vi "Auto_Routine_StraightTwoPieceTRAJ.vi"(8 "error in (no error)":errorcluster) -> (0 "error out":errorcluster)   [LabVIEW 2023]
doc: "Moves from middle of the speaker to the middle note on robot starting line and back \n*****DOES NOT HAVE WAIT AFTER COMPLETE*****\n-Sets arm to speaker Pose\n-Pre rev\n-Waits for arm (to get to speaker shooot pose)\n-Shoots note\n-Waits for box to shoot note\n-Sets arm to floor\n-Runs intake\n-Moves to note\n-Sets arm to speaker pose\n-20 ms wait\n-Goes back to speaker (while waiting for note to intake and pre rev-ing)\n-Waits for arm (to be at speaker shoot pose)\n-Shoots note\n-Waits for shoot to be done \n-Sets arm to floor"
uses:
  Shoulder/ShoulderGetSetpointEnum.ctl
  Trajectory/TrajectoryGlobals.vi
  <vilib>/Rock Robotics/WPI/ThirdParty/JAS_Junk/TrajLib/Trajectory_Library.lvlib
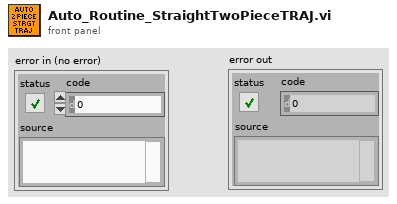
[diagram p1: front panel]
types:
  T1 = typedef "ShoulderGetSetpointEnum.ctl" = enum16{"ShoulderRest", "ShoulderSpeaker", "ShoulderAmp"}
  T2 = typedef "Trajectory_Library.lvlib/TRAJECTORY.ctl" = cluster{"TotalTImeSecs":dbl, "States":T3[]}
  T3 = typedef "Trajectory_Library.lvlib/TRAJ_STATE.ctl" = cluster{"TimeSeconds":dbl, "Velocity":dbl, "Acceleration":dbl, "POSE":T4, "Curvature":dbl}
  T4 = typedef "Trajectory_Library.lvlib/POSE2D.ctl" = cluster{"TRANSLATION":T5, "ROTATION":T6}
  T5 = typedef "Trajectory_Library.lvlib/TRANSLATION2D.ctl" = cluster{"X":dbl, "Y":dbl}
  T6 = typedef "Trajectory_Library.lvlib/ROTATION2D.ctl" = cluster{"VALUE":dbl, "COS":dbl, "SIN":dbl}
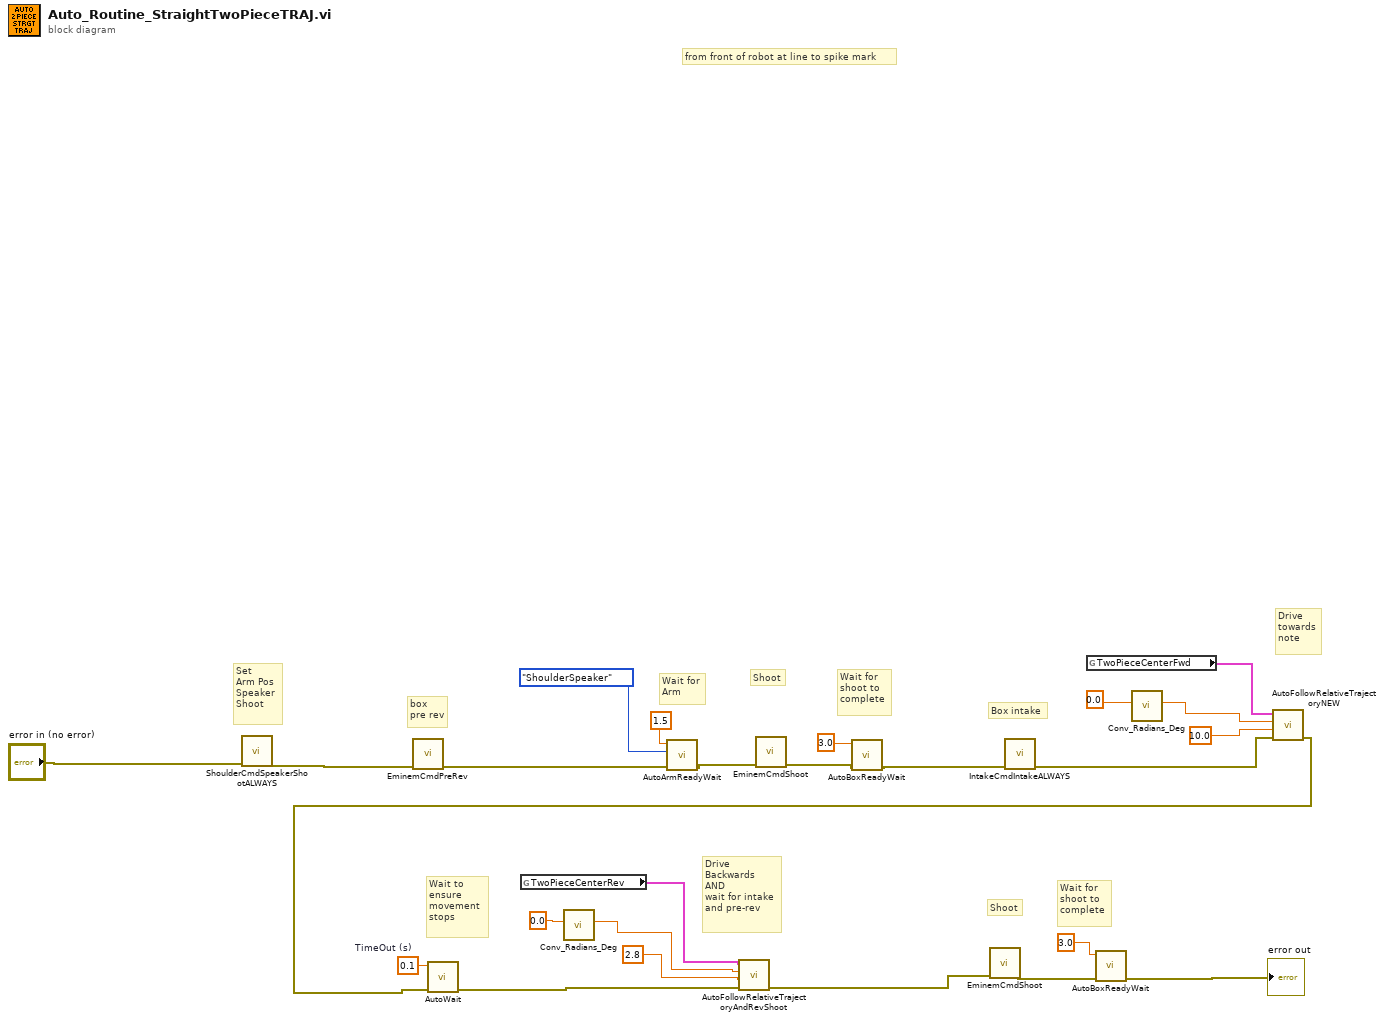
[diagram p0: block diagram]
diagram:
  w8 = 0.1  # TimeOut (s)
  # "Wait to\nensure \nmovement\nstops"
  # "Wait for\nshoot to\ncomplete"
  # "Shoot"
  # "Drive\nBackwards\nAND\nwait for intake\nand pre-rev"
  # "Drive\ntowards\nnote"
  # "box \npre rev"
  # "Box intake"
  # "Wait for\nshoot to\ncomplete"
  # "Shoot"
  # "Wait for\nArm"
  # "Set\nArm Pos\nSpeaker\nShoot"
  # "from front of robot at line to spike mark"
  n1 = call "ShoulderCmdSpeakerShootALWAYS.vi"("error in (no error)"="error in (no error)") -> ("error out"=w16:errorcluster)  [unwired: 10 in]
  n2 = call "EminemCmdPreRev.vi"("error in"=w16) -> ("error out"=w17:errorcluster)  [unwired: 10 in]
  n3 = global read "TrajectoryGlobals.vi" "TwoPieceCenterRev"() -> (w12:T2)
  n4 = call <vilib>:"Conv_Radians_Deg.vi"("Radians"=0.0) -> ("Degrees"=w11:dbl)  [unwired: 10 in]
  n5 = call "AutoArmReadyWait.vi"("error in (no error)"=w17, "ArmSetpoints"=ShoulderGetSetpointEnum."ShoulderSpeaker", "TimeOut (s)"=1.5) -> ("error out"=w22:errorcluster)  [unwired: 8 in]
  n6 = call "EminemCmdShoot.vi"("error in (no error)"=w22) -> ("error out"=w24:errorcluster)  [unwired: 10 in]
  n7 = call "AutoBoxReadyWait.vi"("error in (no error)"=w24, "TimeOut (s)"=3.0) -> ("error out"=w2:errorcluster)  [unwired: 9 in]
  n8 = call "IntakeCmdIntakeALWAYS.vi"("error in (no error)"=w2) -> ("error out"=w1:errorcluster)  [unwired: 10 in]
  n9 = global read "TrajectoryGlobals.vi" "TwoPieceCenterFwd"() -> (w21:T2)
  n10 = call <vilib>:"Conv_Radians_Deg.vi"("Radians"=0.0) -> ("Degrees"=w19:dbl)  [unwired: 10 in]
  n11 = call "AutoFollowRelativeTrajectoryNEW.vi"("error in (no error)"=w1, "TimeOut (s)"=10.0, "End Orientation"=w19, "Trajectory"=w21) -> ("error out"=w6:errorcluster)  [unwired: 7 in]
  n12 = call "AutoWait.vi"("error in (no error)"=w6, "TimeOut (s)"=w8) -> ("error out"=w9:errorcluster)  [unwired: 9 in]
  n13 = call "AutoFollowRelativeTrajectoryAndRevShoot.vi"("error in (no error)"=w9, "TimeOut (s)"=2.8, "End Orientation"=w11, "Trajectory"=w12) -> ("error out"=w5:errorcluster)  [unwired: 7 in]
  n14 = call "EminemCmdShoot.vi"("error in (no error)"=w5) -> ("error out"=w14:errorcluster)  [unwired: 10 in]
  n15 = call "AutoBoxReadyWait.vi"("error in (no error)"=w14, "TimeOut (s)"=3.0) -> ("error out"=→"error out":errorcluster)  [unwired: 9 in]
